vi "Config - Update.vi"(8 "error in (no error)":errorcluster, 10 "Config Data":T1, 11 "Config Data Array":T1[](array[typedef])) -> (0 "error out":errorcluster, 3 "Config Data Array":T1[](array[typedef]))   [LabVIEW 2017]
doc: "Provides update mechanism for the configuration data records."
uses:
  Controls/Config Data.ctl
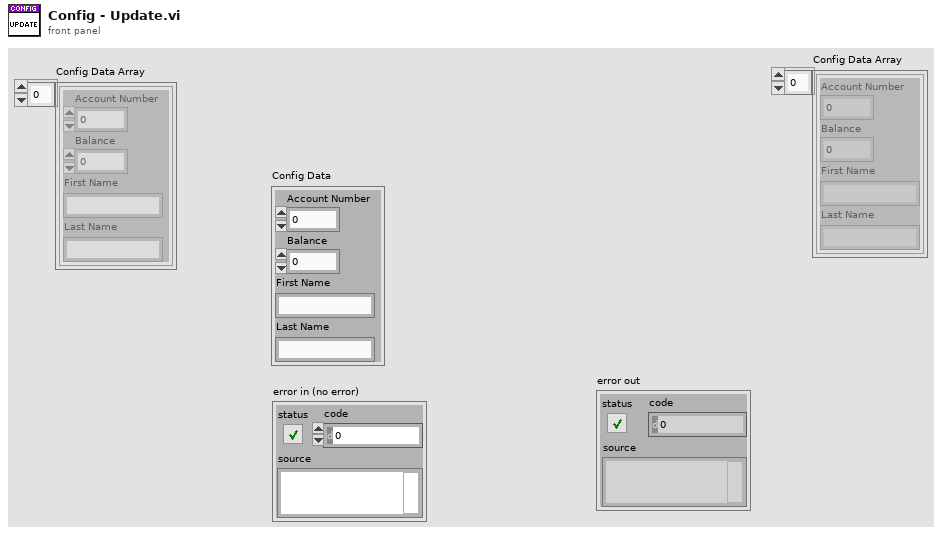
[diagram p1: front panel]
types:
  T1 = typedef "Config Data.ctl" = cluster{"Account Number":i32, "Balance":dbl, "First Name":string, "Last Name":string}
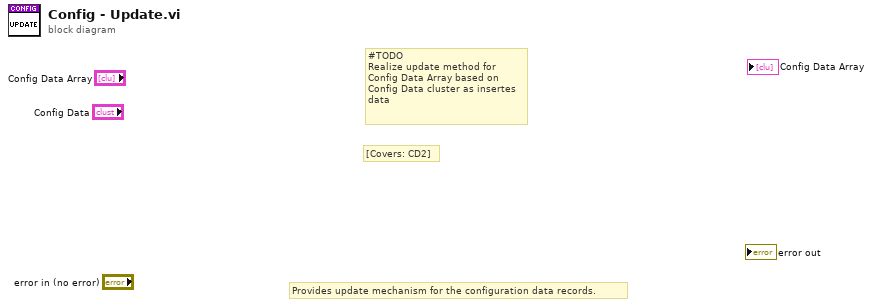
[diagram p0: block diagram]
diagram:
  # "Provides update mechanism for the configuration data records."
  # "[Covers: CD2]"
  # "#TODO\nRealize update method for\nConfig Data Array based on \nConfig Data cluster as insertes\ndata"
